vi "MAIN_close_scan_FPGA.vi"(0 "Sample name":string="RAMM_Test", 1 "Saving path":path=path "C:/Users/sCMOS-1/Desktop/DATA", 2 "queue piezo":refnum<queue>, 3 "queue ASI stage":refnum<queue>, 4 "queue CAMERA":refnum<queue>, 5 "Laser list Refnum":refnum<vi>, 6 "queue FPGA":refnum<queue>, 7 "Illumination source":bool, 9 "Start acquisition":bool, 11 "Measure QPD":bool, 12 "error in":errorcluster, 13 "Global parameters":T1 {"# repetitions" min=0; "Dt (s)" min=0 step=1; "Filter list" items=["ET665lp", "zet405/488/561/640m", "None", "None", "None", "None"]}) -> (8 "Next task":T2, 14 "error out":errorcluster)   [LabVIEW 2015]
uses:
  CONTROLS/Q_main_element.ctl
  CONTROLS/Global parameters.ctl
  CONTROLS/Q_MCL_piezo_element.ctl
  CONTROLS/Q_ASI_stage_element.ctl
  CONTROLS/Q_camera_element.ctl
  CONTROLS/Q_FPGA_element.ctl
  GLOBAL/Global_MAIN.vi
  GLOBAL/Global_ABORT.vi
panel:
  out "Laser lines manager":i32(listbox)=-1
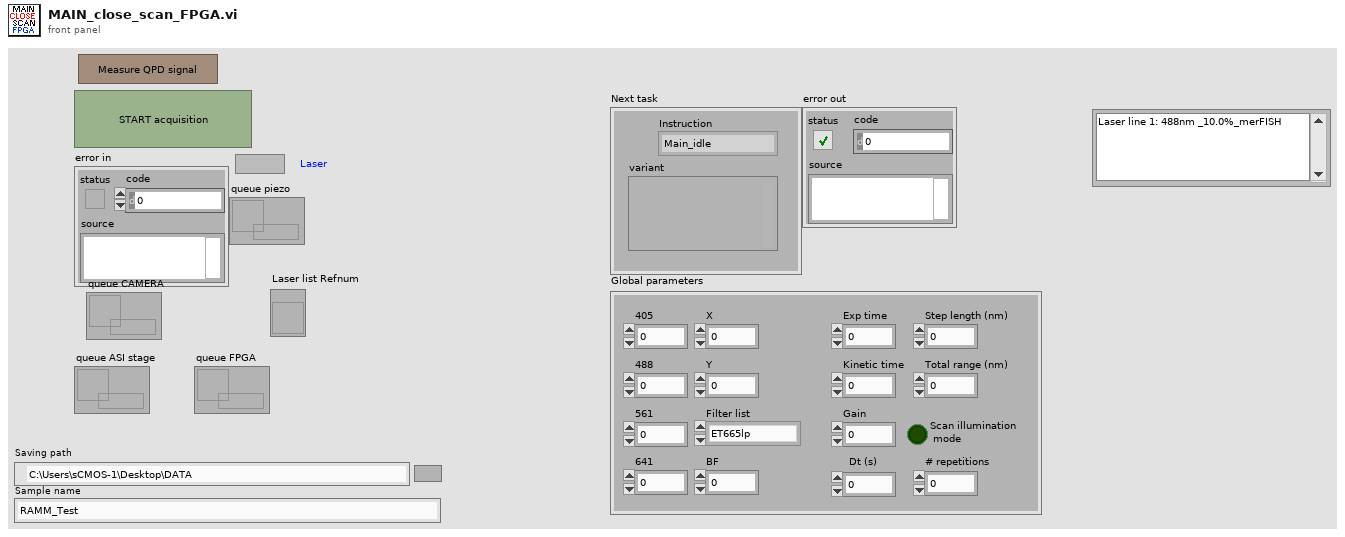
[diagram p1: front panel]
types:
  T1 = typedef "Global parameters.ctl" = cluster{"405":dbl, "488":dbl, "561":dbl, "641":dbl, "BF":dbl, "X":dbl, "Y":dbl, "Filter list":u16, "Exp time":sgl, "Kinetic time":sgl, "Gain":i32, "Step length (nm)":u32, "Total range (nm)":u32, "Scan illumination\n mode":bool, "Dt (s)":i32, "# repetitions":i32}
  T2 = typedef "Q_main_element.ctl" = cluster{"variant":variant, "Instruction":enum16{"Main_idle", "Main_initialize", "Main_initialize_TDMS", "Main_initialize_Queue", "Main_error", "Main_DAQ_initialization_results", "Main_ASI_initialization_results", "Main_Piezo_initialization_results", "Main_Valve_initialization_results", "Main_Pump_initialization_results", "Main_CAMERA_initialization_results", "Main_FPGA_initialization_results", "Main_DAQ_error", "Main_ASI_error", "Main_Piezo_error", "Main_CAMERA_error", "Main_Valve_error", "Main_Pump_error", "Main_FPGA_error", "Main_start_acquiring", "Main_not_acquiring", "Main_acquiring", "Main_stop_acquiring", "Main_change_exposure", "Main_change_z_scan_parameters", "Main_define_ROI", "Main_define_mosaic", "Main_read_kinetic_time", "Main_cooler", "Main_read_temperature", "Main_save_XY", "Main_load_XY", "Main_discard_XY", "Main_move_to_XY", "Main_measure_QPD", "Main_autofocus_calibration", "Main_autofocus_initialization", "Main_autofocus_stop", "Main_save_PID", "Main_change_H_valve_position", "Main_two_way_valve", "Main_save_movie", "Main_init_single_scan", "Main_single_scan", "Main_stop_single_scan", "Main_merFISH_illumination_parameters", "Main_merFISH_buffer_probe_list", "Main_merFISH_injections_procedure", "Main_merFISH_save_setpoint", "Main_merFISH_DAPI_parameters", "Main_merFISH_Brightfield_parameters", "Main_merFISH_save_embryo_ROI", "Main_merFISH_init", "Main_merFISH_resume", "Main_merFISH_start_autofocus", "Main_merFISH_open_close_valve_merFISH", "Main_merFISH_open_close_valve_photobleaching", "Main_merFISH_hybridization", "Main_merFISH_move_to_ROI", "Main_merFISH_wait_stabilization", "Main_merFISH_move_to_REF", "Main_merFISH_scan", "Main_merFISH_photobleaching_injection", "Main_merFISH_photobleaching", "Main_merFISH_send_email", "Main_merFISH_close", "Main_STOP"}}
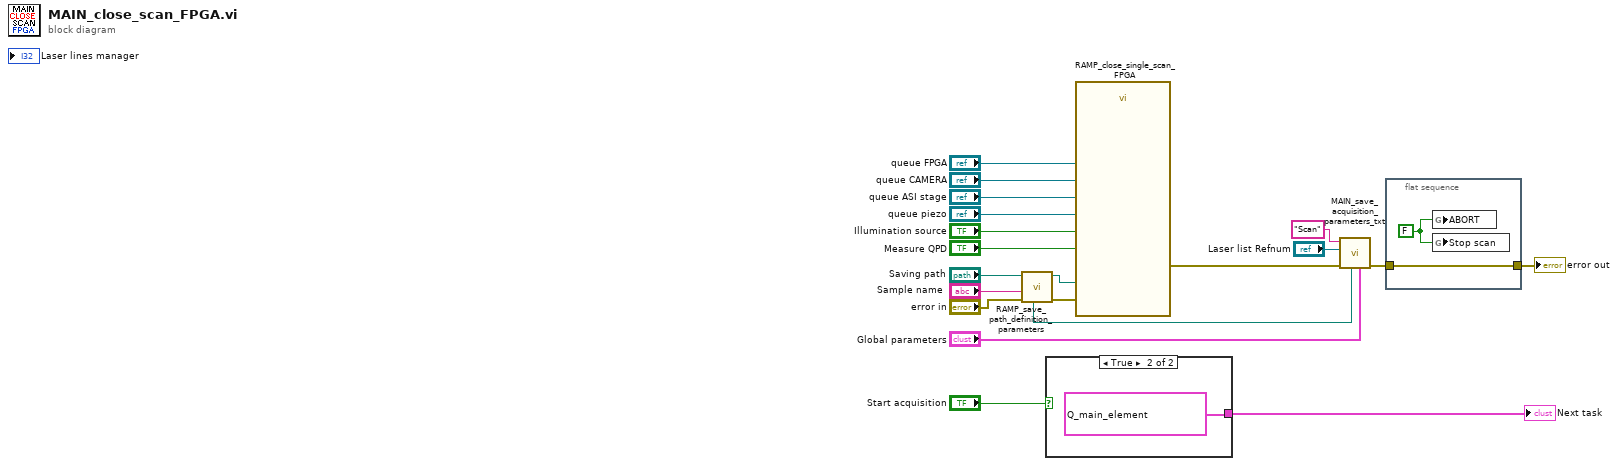
[diagram p0: block diagram]
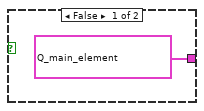
[diagram p2: hidden frame]
diagram:
  n1 = call "RAMP_save_path_definition_parameters.vi"("error in"="error in", "Sample name"="Sample name", "Path to the saving folder"="Saving path") -> ("error out"=w16:errorcluster, "Z_position_file path"=w20:path, "Acquisition_parameters path"=w19:path)  [unwired: 3 in]
  n2 = case shown="True" "Start acquisition" {
    tunnel: [T2 {"variant"=variant, "Instruction"=enum."Main_not_acquiring"} ("Q_main_element") T2 {"variant"=variant, "Instruction"=enum."Main_start_acquiring"} ("Q_main_element")] -> w14
    frame False {
    }
    frame True {
    }
  }
  "Next task" <- w14
  n3 = call "RAMP_close_single_scan_FPGA.vi"("queue FPGA"="queue FPGA", "queue ASI stage"="queue ASI stage", "queue CAMERA"="queue CAMERA", "Measure QPD"="Measure QPD", "queue piezo"="queue piezo", "error in"=w16, "Z_position_file path"=w20, "Illumination source"="Illumination source") -> ("error out"=w17:errorcluster)  [unwired: 7 in]
  n4 = call "MAIN_save_acquisition_parameters_txt.vi"("Global parameters"="Global parameters", "file path"=w19, "error in"=w17, "Laser list Refnum"="Laser list Refnum", "Data type"="Scan") -> ("error out"=w3:errorcluster)  [unwired: 6 in]
  n5 = flat-sequence {
    tunnel: w3 -> [w24]
    tunnel: [w24] -> w2
    frame #0 {
      w23 = FALSE ("Abort scan")
      n6 = global write "Global_ABORT.vi" "ABORT"(w23) -> ()
      n7 = global write "Global_MAIN.vi" "Stop scan"(w23) -> ()
    }
  }
  "error out" <- w2
